vi "Read Class Name.vi"(8 "error in (no error)":errorcluster, 11 "Ctrl Reference's in":refnum<class "Ctrl Reference's.lvclass">) -> (0 "error out":errorcluster, 2 "Class Name":string, 3 "Ctrl Reference's out":refnum<class "Ctrl Reference's.lvclass">)   [LabVIEW 2020, in "Ctrl Reference's.lvclass"]
uses:
  Ctrl Reference's.lvclass
  Ctrl Reference's.lvclass/Ctrl Reference's.ctl
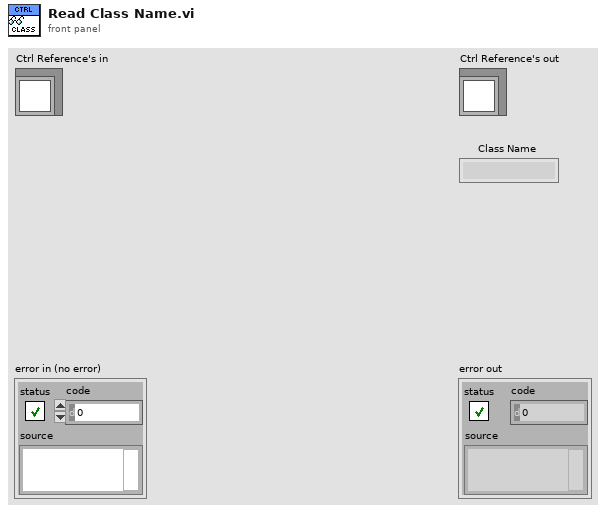
[diagram p1: front panel]
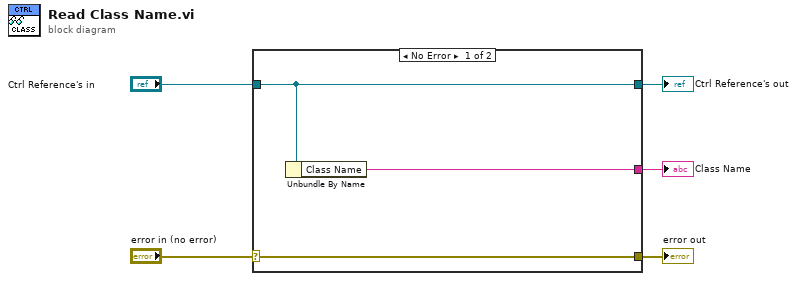
[diagram p0: block diagram]
diagram:
  n1 = case shown="No Error" "error in (no error)" {
    selector: "error in (no error)" -> [w8 w9]
    tunnel: [w8 w9] -> w4
    tunnel: [w7 w10] -> w2
    tunnel: "Ctrl Reference's in" -> [w7 w10]
    tunnel: [w6 _] -> w1
    frame No Error {
      n2 = Unbundle By Name(w7) -> ("Class Name"=w6:string)
    }
    frame Error {
    }
  }
  "error out" <- w4
  "Ctrl Reference's out" <- w2
  "Class Name" <- w1
